vi "Apply Gradient Power Supply.vi"(8 "Reminder":dbl, 9 "Setpoint":dbl, 10 "Gradient":dbl=-1000.0 format="%#_13g", 11 "Iteration Interval":dbl=0.01 format="%#_13g") -> (3 "Current Setpoint":dbl)   [LabVIEW 2023]
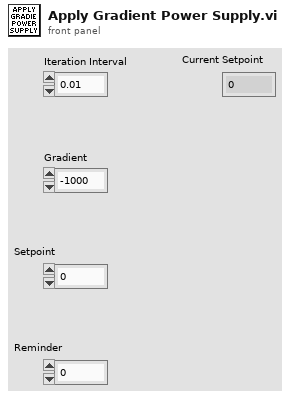
[diagram p1: front panel]
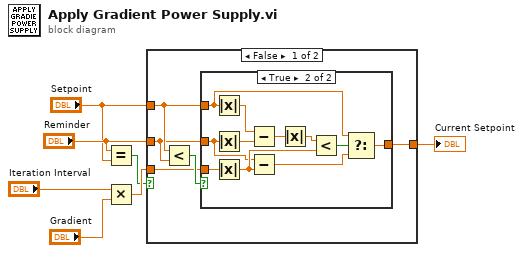
[diagram p0: block diagram]
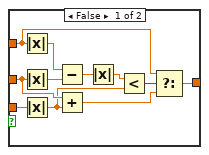
[diagram p2: hidden frame]
diagram:
  n1 = Equal?(x="Reminder", y="Setpoint") -> (x = y?=w2:bool)
  n2 = Multiply(x="Iteration Interval", y="Gradient") -> (x*y=w7:dbl)
  n3 = case shown="False" w2 {
    tunnel: [w8 w35] -> w4
    tunnel: "Setpoint" -> [w11 w35]
    tunnel: "Reminder" -> [w10 _]
    tunnel: w7 -> [w9 _]
    frame False {
      n4 = Less?(x=w11, y=w10) -> (x < y?=w12:bool)
      n5 = case shown="True" w12 {
        tunnel: w11 -> [w15 w25]
        tunnel: w10 -> [w18 w27]
        tunnel: w9 -> [w23 w34]
        tunnel: [w13 w24] -> w8
        frame False {
          n6 = Absolute Value(x=w15) -> (abs(x)=w21:dbl)
          n7 = Absolute Value(x=w18) -> (abs(x)=w22:dbl)
          n8 = Absolute Value(x=w23) -> (abs(x)=w17:dbl)
          n9 = Subtract(x=w21, y=w22) -> (x-y=w20:dbl)
          n10 = Add(x=w18, y=w17) -> (x+y=w16:dbl)
          n11 = Absolute Value(x=w20) -> (abs(x)=w19:dbl)
          n12 = Less?(x=w19, y=w17) -> (x < y?=w14:bool)
          n13 = Select(t=w15, s=w14, f=w16) -> (s? t:f=w13:dbl)
        }
        frame True {
          n14 = Absolute Value(x=w25) -> (abs(x)=w32:dbl)
          n15 = Absolute Value(x=w27) -> (abs(x)=w33:dbl)
          n16 = Absolute Value(x=w34) -> (abs(x)=w28:dbl)
          n17 = Subtract(x=w32, y=w33) -> (x-y=w31:dbl)
          n18 = Subtract(x=w27, y=w28) -> (x-y=w26:dbl)
          n19 = Absolute Value(x=w31) -> (abs(x)=w30:dbl)
          n20 = Less?(x=w30, y=w28) -> (x < y?=w29:bool)
          n21 = Select(t=w25, s=w29, f=w26) -> (s? t:f=w24:dbl)
        }
      }
    }
    frame True {
    }
  }
  "Current Setpoint" <- w4
